vi "get_readiness.vi"(8 "error in (no error)":errorcluster, 11 "GenericDAQ in":refnum<class "GenericDAQ.lvclass">) -> (0 "error out":errorcluster, 2 "ready?":bool=TRUE, 3 "GenericDAQ out":refnum<class "GenericDAQ.lvclass">)   [LabVIEW 2010, in "GenericDAQ.lvclass"]
uses:
  GenericDAQ.lvclass
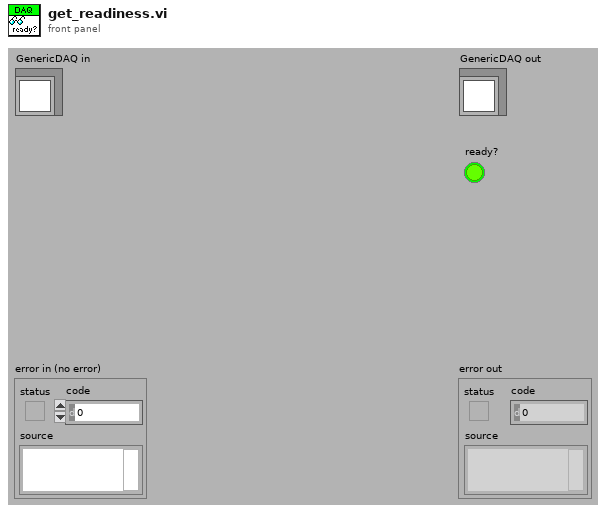
[diagram p1: front panel]
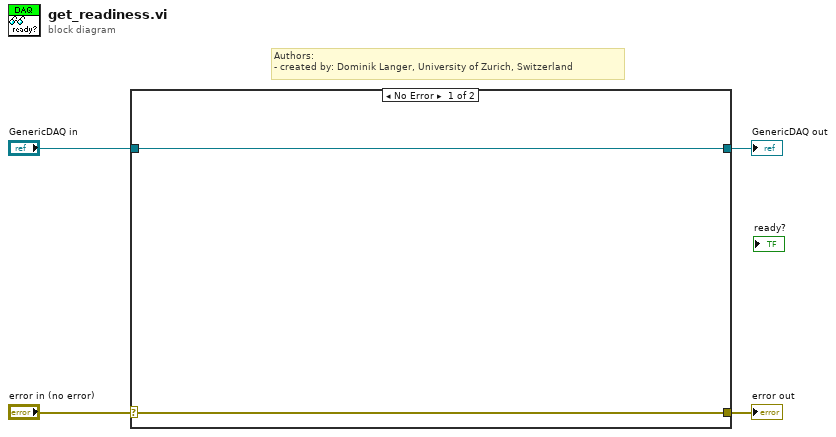
[diagram p0: block diagram]
diagram:
  # "Authors: \n- created by: Dominik Langer, University of Zurich, Switzerland"
  n1 = case shown="No Error" "error in (no error)" {
    selector: "error in (no error)" -> [w5 w8]
    tunnel: [w5 w8] -> w3
    tunnel: [w6 w7] -> w1
    tunnel: "GenericDAQ in" -> [w6 w7]
    frame No Error {
    }
    frame Error {
    }
  }
  "error out" <- w3
  "GenericDAQ out" <- w1
